vi "Split Lines.vi"(8 "error in (no error)":errorcluster, 10 "spreadsheet string":string, 11 "Construct String Header in":refnum<class "Construct String Header.lvclass">) -> (0 "error out":errorcluster, 2 "array":string[](array[string]), 3 "Construct String Header out":refnum<class "Construct String Header.lvclass">)   [LabVIEW 2018, in "Construct String Header.lvclass"]
doc: "Este VI recebe uma string e retorna um array onde cada elemento cotém uma das linhas da string."
uses:
  Construct String Header.lvclass
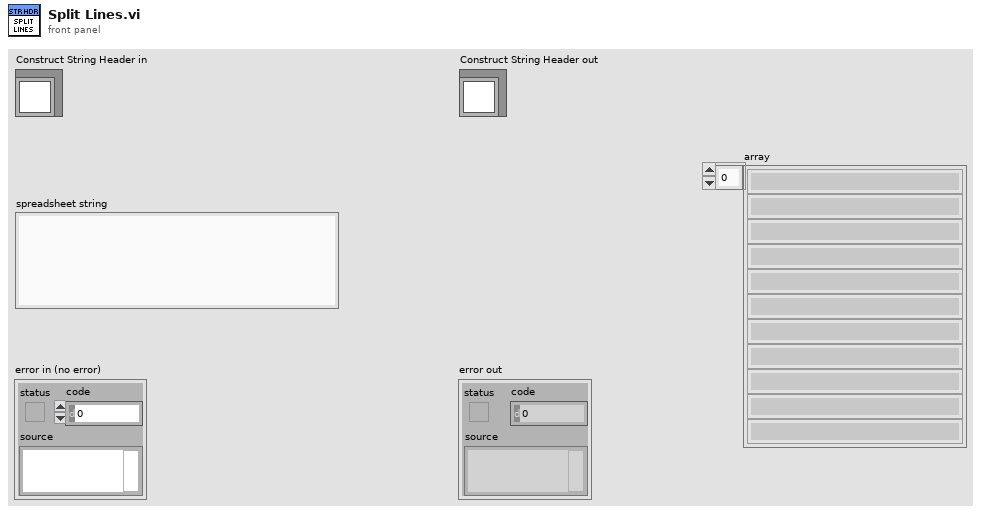
[diagram p1: front panel]
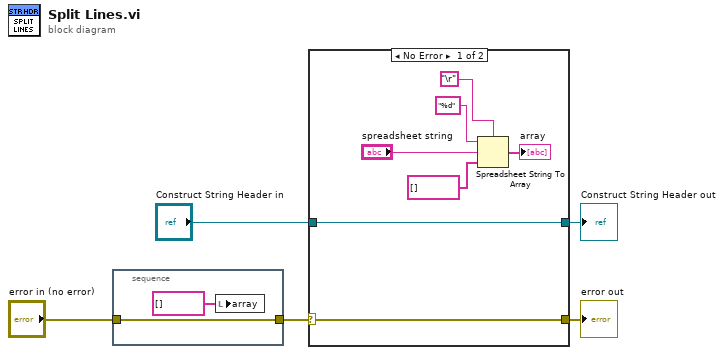
[diagram p0: block diagram]
diagram:
  n1 = stacked-sequence {
    tunnel: "error in (no error)" -> [w6]
    tunnel: [w6] -> w1
    frame #0 {
      n2 = local write "array"(string[] []) -> ()
    }
  }
  n3 = case shown="No Error" w1 {
    selector: w1 -> [w13 w16]
    tunnel: [w13 w16] -> w3
    tunnel: [w14 w15] -> w4
    tunnel: "Construct String Header in" -> [w14 w15]
    frame No Error {
      n4 = Spreadsheet String To Array(delimiter (Tab)="\r", format string="%d", spreadsheet string="spreadsheet string", array type (2D Dbl)=string[] []) -> (array=→"array":string[])
    }
    frame Error {
    }
  }
  "error out" <- w3
  "Construct String Header out" <- w4
